vi "Write FGV Data.vi"(0 "Station Action in":refnum<class "Station Action.lvclass">, 1 "0Cv/1St":i32, 5 "DataIn":string, 7 "Data":T1=enum."CurrentAction", 11 "error in (no error)":errorcluster) -> (4 "Station Action out":refnum<class "Station Action.lvclass">, 15 "error out":errorcluster)   [LabVIEW 2019, in "Station Action.lvclass"]
uses:
  Station Action.lvclass
  Ctrl/Auto Inspection Data Name.ctl
  Ctrl/Auto Inspection Station Name2.ctl
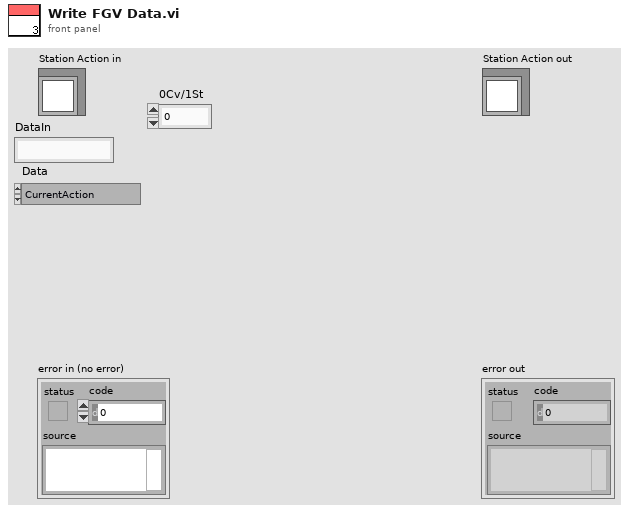
[diagram p1: front panel]
types:
  T1 = typedef "Auto Inspection Data Name.ctl" = enum16{"LocalRun", "ItemSN(TimeCode)", "CurrentAction", "Error", "Data", "OKNG", "電壓值", "電壓值判斷", "電流值", "電流值判斷", "Laser1 Data", "Laser2 Data", "Laser OKNG", "StationNO"}
  T2 = typedef "Auto Inspection Station Name2.ctl" = enum16{"S1Barcode", "S2Measure", "S3Measure", "S4Measure", "S5Measure", "S11_LaserCheck", "S8_Vision AI"}
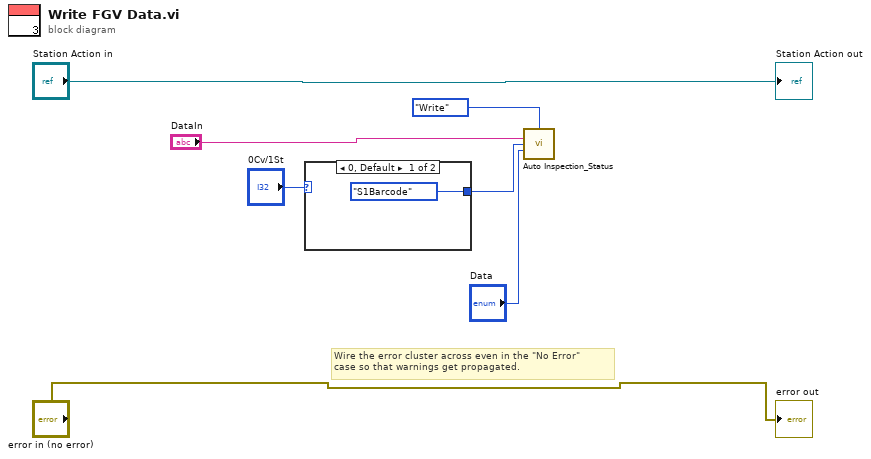
[diagram p0: block diagram]
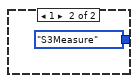
[diagram p2: hidden frame]
diagram:
  # "Wire the error cluster across even in the \"No Error\"\ncase so that warnings get propagated."
  n1 = case shown="0, Default" "0Cv/1St" {
    tunnel: [Auto_Inspection_Station_Name2."S1Barcode" ("Station") Auto_Inspection_Station_Name2."S3Measure" ("Station")] -> w4
    frame 0, Default {
    }
    frame 1 {
    }
  }
  n2 = call "Auto Inspection_Status.vi"("Action"=enum16{"Initial", "Write", "Read"}."Write", "DataIn"="DataIn", "Station"=w4, "Data"="Data") -> ()  [unwired: 9 in, 3 out]
  "error out" <- "error in (no error)"
  "Station Action out" <- "Station Action in"
